vi "ROI entry-Shortcut menus handler.vi"(11 "ItemTag":string) -> ()   [LabVIEW 2017]
uses:
  Typedefs/ROI management FG states.ctl
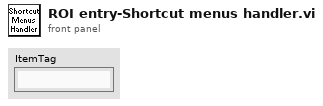
[diagram p1: front panel]
types:
  T1 = typedef "ROI management FG states.ctl" = enum16{"Read", "Write", "Clear Last", "Clear All", "Update ROIs time", "Reload last ROI set", "Offset all ROI", "Offset visible ROI"}
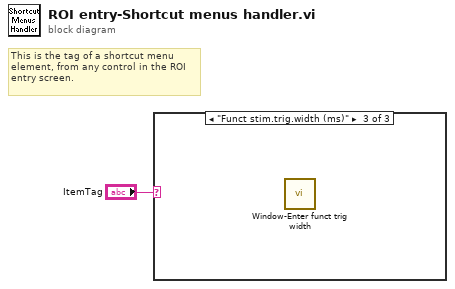
[diagram p0: block diagram]
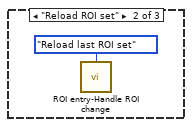
[diagram p3: hidden frame]
diagram:
  # "This is the tag of a shortcut menu element, from any control in the ROI entry screen."
  n1 = case shown="\"Funct stim.trig.width (ms)\"" "ItemTag" {
    frame Default {
    }
    frame "Reload ROI set" {
      n2 = call "ROI entry-Handle ROI change.vi"("ROI management"=ROI_management_FG_states."Reload last ROI set" ("Function")) -> ()  [unwired: 8 in, 3 out]
    }
    frame "Funct stim.trig.width (ms)" {
      n3 = call "Window-Enter funct trig width.vi"() -> ()  [unwired: 11 in, 1 out]
    }
  }
